vi "IK_Err.vi"(2 "Current Pose":T1, 3 "Target Pose":T1) -> (1 "error":dbl[](array[numeric]))   [LabVIEW 2024]
uses:
  <vilib>/Analysis/Matrix/Datatypes/RealMatrix.ctl
  <vilib>/Analysis/NI_AALPro.lvlib
  <vilib>/Analysis/Matrix/NI_Matrix.lvlib
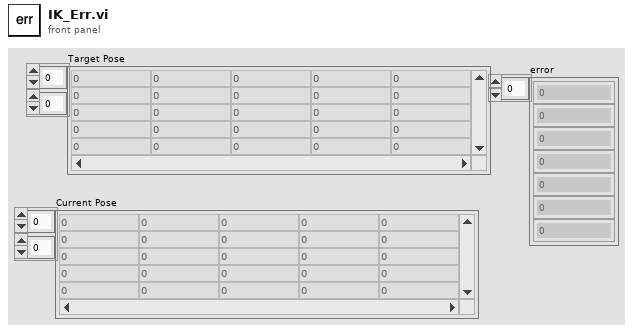
[diagram p1: front panel]
types:
  T1 = typedef "NI_Matrix.lvlib/RealMatrix.ctl" = dbl[][]
  T2 = typedef "NI_Kinematics.lvlib/Quaternion.ctl" = dbl[]
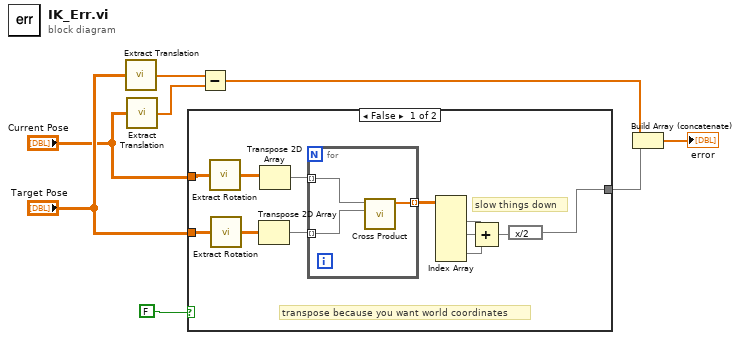
[diagram p0: block diagram]
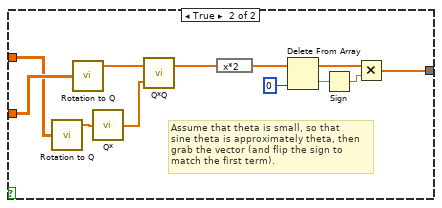
[diagram p2: hidden frame]
diagram:
  n1 = call <userlib>:"Extract Translation.vi"("Transformation matrix"="Target Pose") -> ("Position"=w8:dbl[])
  n2 = call <userlib>:"Extract Translation.vi"("Transformation matrix"="Current Pose") -> ("Position"=w7:dbl[])
  n3 = case shown="False" FALSE {
    tunnel: "Target Pose" -> [w9 w26]
    tunnel: "Current Pose" -> [w10 w25]
    tunnel: [w11 w24] -> w2
    frame False {
      # "slow things down"
      # "transpose because you want world coordinates"
      n4 = call <userlib>:"Extract Rotation.vi"("Transformation matrix"=w10) -> ("Rotation matrix"=w18:T1)
      n5 = call <userlib>:"Extract Rotation.vi"("Transformation matrix"=w9) -> ("Rotation matrix"=w17:T1)
      n6 = Transpose 2D Array(2D array=w17) -> (transposed array=w19:T1)
      n7 = Transpose 2D Array(2D array=w18) -> (transposed array=w20:T1)
      n8 = for {
        tunnel: w19 -> [w21] mode=indexing
        tunnel: w20 -> [w22] mode=indexing
        tunnel: [w23] -> w12 mode=indexing
        n9 = call <vilib>:"Cross Product.vi"("B Vector"=w21, "A Vector"=w22) -> ("Cross Product"=w23:dbl[])  [unwired: 8 in, 1 out]
      }
      n10 = Index Array(array=w12) -> (element #1=w15:dbl[], element #2=w14:dbl[], element #3=w13:dbl[])  [unwired: 6 in]
      n11 = Compound Arithmetic op=ADD(w15, w14, w13) -> (w16:dbl[])
      n12 = expression code="x/2"(w16) -> (w11:dbl[])
    }
    frame True {
      # "Assume that theta is small, so that \nsine theta is approximately theta, then\ngrab the vector (and flip the sign to \nmatch the first term)."
      n13 = call <userlib>:"Rotation to Q.vi"("Rotation matrix"=w25) -> ("quaternion"=w29:dbl[])  [unwired: 2 out]
      n14 = call <userlib>:"Rotation to Q.vi"("Rotation matrix"=w26) -> ("quaternion"=w28:dbl[])  [unwired: 2 out]
      n15 = call <userlib>:"Q*.vi"("quaternion"=w29) -> ("quaternion*"=w30:T2)
      n16 = call <userlib>:"Q*Q.vi"("quaternion B"=w30, "quaternion A"=w28) -> ("AxB"=w27:dbl[])  [unwired: 1 out]
      n17 = expression code="x*2"(w27) -> (w35:dbl[])
      n18 = Delete From Array(array=w35, index=0) -> (deleted portion=w32:dbl, array with subset deleted=w34:dbl[])  [unwired: 1 in]
      n19 = Sign(1:w32) -> (0:w33:dbl)
      n20 = Multiply(x=w34, y=w33) -> (x*y=w24:dbl[])
    }
  }
  n21 = Subtract(x=w8, y=w7) -> (x-y=w5:dbl[])
  n22 = Build Array (concatenate)(w5, w2) -> (→"error":dbl[])
